vi "Global Variable Monitor.vi"() -> ()   [LabVIEW 2018, in "ASIA Pump.lvlib"]
uses:
  ASIA Pump.lvlib
panel:
  out "ASIA Pump Global":T1(array[cluster])
  in  "stop":bool
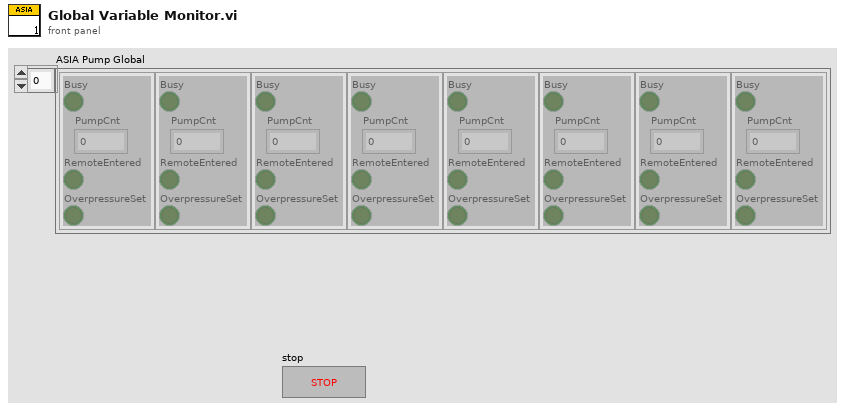
[diagram p1: front panel]
types:
  T1 = cluster{"Busy":bool, "PumpCnt":dbl, "RemoteEntered":bool, "OverpressureSet":bool}[]
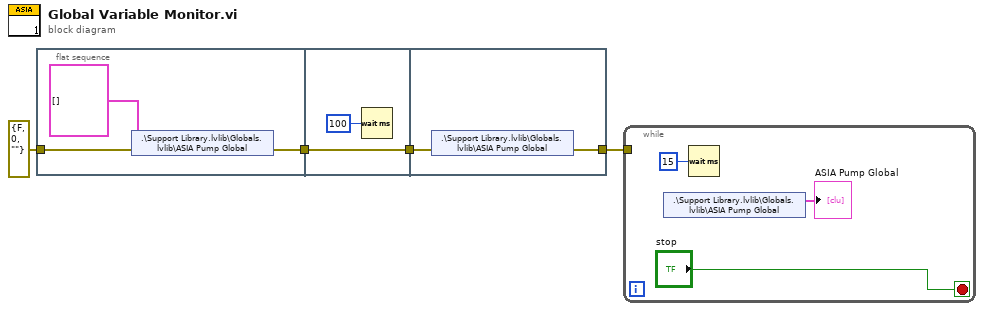
[diagram p0: block diagram]
diagram:
  n1 = flat-sequence {
    tunnel: [w7] -> w4
    tunnel: errorcluster {"status"=FALSE, "code"=0, "source"=""} ("error in (no error)") -> [w6]
    tunnel: w4 -> [w9]
    tunnel: [w9] -> w3
    tunnel: w3 -> [w11]
    tunnel: [w10] -> w2
    frame #0 {
      n2 = shared-variable ".\\Support Library.lvlib\\Globals.lvlib\\ASIA Pump Global"(T1 [] ("ASIA Pump Global"), error in=w6) -> (error out=w7:errorcluster)
    }
    frame #1 {
      n3 = Wait (ms)(milliseconds to wait=u32 100) -> ()  [unwired: 1 out]
    }
    frame #2 {
      n4 = shared-variable ".\\Support Library.lvlib\\Globals.lvlib\\ASIA Pump Global"(error in=w11) -> (error out=w10:errorcluster)  [unwired: 1 out]
    }
  }
  n5 = while {
    tunnel: w2 -> [_]
    stop <- "stop" stop-if-true
    n6 = shared-variable ".\\Support Library.lvlib\\Globals.lvlib\\ASIA Pump Global"() -> (→"ASIA Pump Global":T1)  [unwired: 1 in, 1 out]
    n7 = Wait (ms)(milliseconds to wait=u32 15) -> ()  [unwired: 1 out]
  }
